vi "Optimize 1D.vi"(5 "AO Channel":tag="Dev1/ao0", 7 "Fit Method":enum16{"Max", "Gaussian"}(ring), 8 "Dwell Time (ms)":i32=2, 9 "Volt Step":dbl, 10 "Volt Range":dbl, 11 "Curr Pos":dbl) -> (3 "Final Pos":dbl)   [LabVIEW 2012]
uses:
  <vilib>/Analysis/NI_AALPro.lvlib
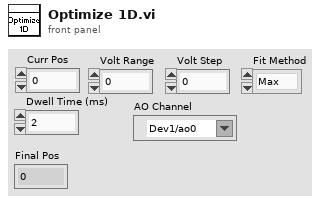
[diagram p1: front panel]
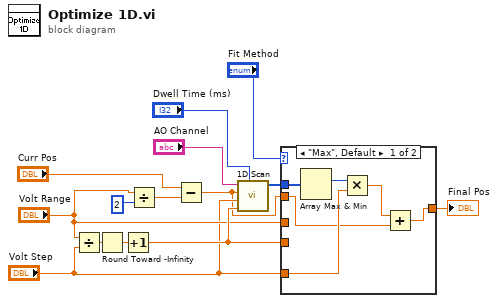
[diagram p0: block diagram]
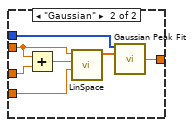
[diagram p2: hidden frame]
diagram:
  n1 = Divide(x="Volt Range", y="Volt Step") -> (x/y=w12:dbl)
  n2 = Round Toward -Infinity(1:w12) -> (0:w13:dbl)
  n3 = Increment(x=w13) -> (x+1=w7:dbl)
  n4 = Divide(x="Volt Range", y=2) -> (x/y=w11:dbl)
  n5 = Subtract(x="Curr Pos", y=w11) -> (x-y=w4:dbl)
  n6 = call "1D Scan.vi"("Dwell Time (ms)"="Dwell Time (ms)", "Num Steps"=w7, "Step"="Volt Step", "Min"=w4, "Channel"="AO Channel") -> ("Counts"=w9:i32[])  [unwired: 6 in]
  n7 = case shown="\"Max\", Default" "Fit Method" {
    tunnel: [w15 w27] -> w1
    tunnel: w9 -> [w19 w26]
    tunnel: "Volt Step" -> [w17 _]
    tunnel: w4 -> [w16 w23]
    tunnel: w7 -> [_ w24]
    tunnel: "Volt Range" -> [_ w22]
    frame "Max", Default {
      n8 = Array Max & Min(array=w19) -> (max index (indices)=w18:i32)  [unwired: 3 out]
      n9 = Multiply(x=w18, y=w17) -> (x*y=w20:dbl)
      n10 = Add(x=w20, y=w16) -> (x+y=w15:dbl)
    }
    frame "Gaussian" {
      n11 = Add(x=w23, y=w22) -> (x+y=w21:dbl)
      n12 = call "LinSpace.vi"("Num Steps"=w24, "Max"=w21, "Min"=w23) -> ("Array"=w25:dbl[])  [unwired: 8 in]
      n13 = call <vilib>:"Gaussian Peak Fit.vi"("Y"=w26, "X"=w25) -> ("center"=w27:dbl)  [unwired: 7 in, 6 out]
    }
  }
  "Final Pos" <- w1
